vi "Handle Error.vi"(8 "error in (no error)":errorcluster, 11 "Task in":refnum<class "Task.lvclass">) -> (0 "error out":errorcluster, 2 "stop actor?":bool=TRUE, 3 "Task out":refnum<class "Task.lvclass">)   [LabVIEW 2020, in "Volatus.lvlib" / "Task.lvclass"]
doc: "(<B>Filename</B>: Actor Framework.lvlib:Actor.lvclass:Handle Error.vi)\n\nDefines how the actor handles an error that occurred while processing a message. By default, this method does nothing except stop the actor."
uses:
  Task.lvclass
  Task.lvclass/Task.ctl
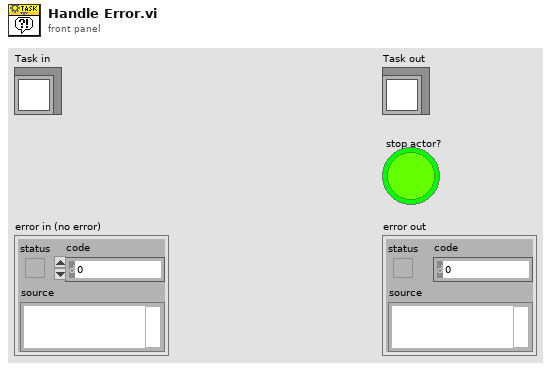
[diagram p1: front panel]
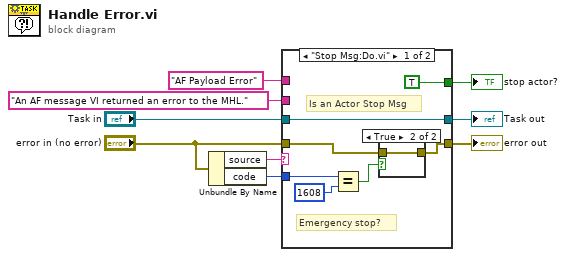
[diagram p0: block diagram]
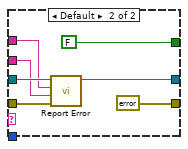
[diagram p3: hidden frame]
diagram:
  n1 = Unbundle By Name("error in (no error)") -> ("source"=w3:string, "code"=w2:i32)
  n2 = case shown="\"Stop Msg:Do.vi\"" w3 {
    tunnel: "error in (no error)" -> [w13 w24]
    tunnel: "Task in" -> [w16 w23]
    tunnel: [w16 w22] -> w7
    tunnel: "AF Payload Error" ("Context") -> [_ w21]
    tunnel: [TRUE ("stop actor?") FALSE ("stop actor?")] -> w5
    tunnel: "An AF message VI returned an error to the MHL." ("Message") -> [_ w19]
    tunnel: w2 -> [w14 _]
    tunnel: [w12 errorcluster {"status"=FALSE, "code"=0, "source"=""} ("error in (no error)")] -> w1
    frame "Stop Msg:Do.vi" {
      # "Emergency stop?"
      # "Is an Actor Stop Msg"
      n3 = Equal?(x=w14, y=1608) -> (x = y?=w10:bool)
      n4 = case shown="True" w10 {
        tunnel: w13 -> [_ w17]
        tunnel: [_ w17] -> w12
        frame False {
        }
        frame True {
        }
      }
    }
    frame Default {
      n5 = call "Report Error.vi"("error in (no error)"=w24, "Message"=w19, "Context"=w21, "Task in"=w23) -> ("Task out"=w22:refnum<class "Task.lvclass">)  [unwired: 6 in, 1 out]
    }
  }
  "Task out" <- w7
  "error out" <- w1
  "stop actor?" <- w5
